vi "complete wheel.vi"(8 "error in (no error)":errorcluster, 10 "number of samples between standards":i32=4, 11 "all rows":string[][](array[string])) -> (0 "error out":errorcluster, 3 "Group run list":string[][](array[string]))   [LabVIEW 2016]
doc: "This vi sorts a wheel list and creates a run order"
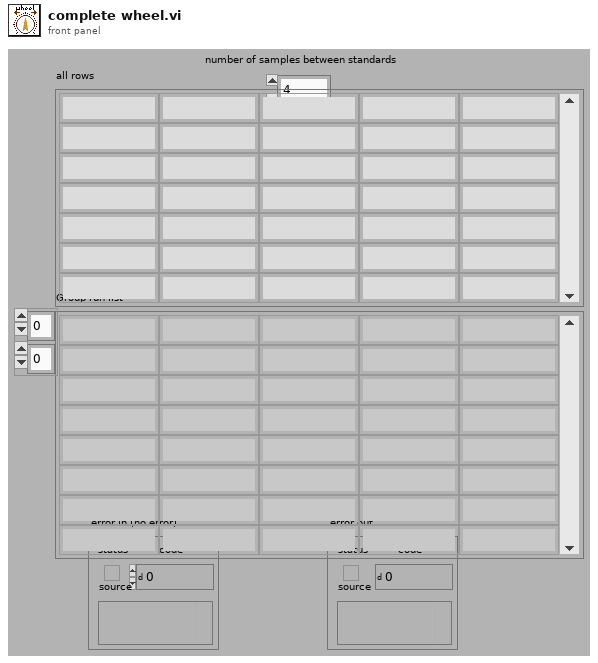
[diagram p1: front panel]
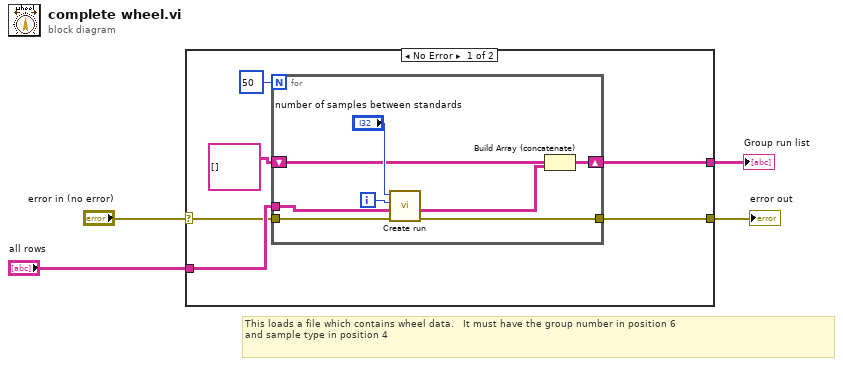
[diagram p0: block diagram]
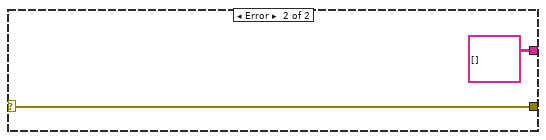
[diagram p2: hidden frame]
diagram:
  # "This loads a file which contains wheel data.   It must have the group number in position 6\nand sample type in position 4"
  n1 = case shown="No Error" "error in (no error)" {
    selector: "error in (no error)" -> [w6 w20]
    tunnel: "all rows" -> [w10 _]
    tunnel: [w9 w20] -> w2
    tunnel: [w5 string[][] []] -> w4
    frame No Error {
      n2 = for {
        N: 50 -> [_]
        tunnel: w10 -> [w18]
        tunnel: w6 -> [w15]
        tunnel: [w14] -> w9
        shift-right: [w12] -> w5
        shift-left: string[][] [] -> [w11]
        i -> [w16]
        n3 = call "Create run.vi"("error in (no error)"=w15, "all rows"=w18, "Which group"=w16, "number of samples between standards"="number of samples between standards") -> ("error out"=w14:errorcluster, "Group run list"=w13:string[][])  [unwired: 6 out]
        n4 = Build Array (concatenate)(w11, w13) -> (w12:string[][])
      }
    }
    frame Error {
    }
  }
  "error out" <- w2
  "Group run list" <- w4
